vi "Serial Init.vi"(8 "error in (no error)":errorcluster, 11 "VISA Refnum in":refnum<visa-resource-name>) -> (0 "error out":errorcluster, 3 "Boolean":bool)   [LabVIEW 2017]
uses:
  <vilib>/Instr/_visa.llb/VISA Configure Serial Port (Instr).vi
  <vilib>/regexp/Match Regular Expression.xnode
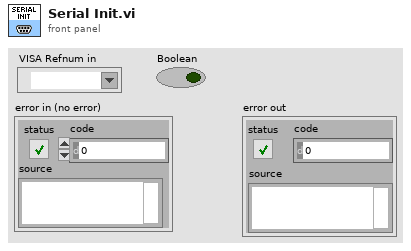
[diagram p1: front panel]
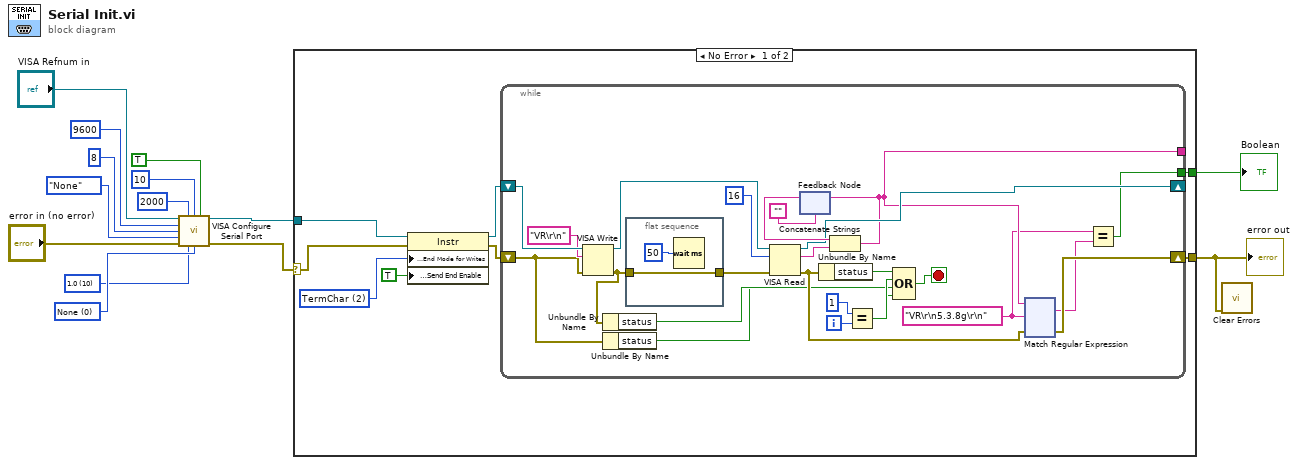
[diagram p0: block diagram]
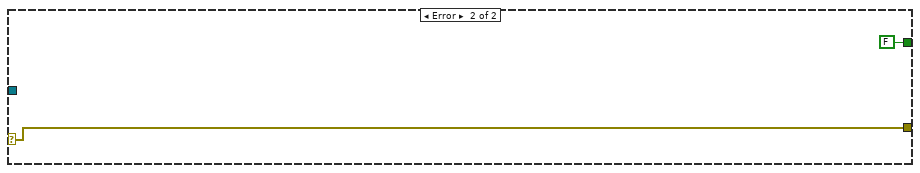
[diagram p2: hidden frame]
diagram:
  w11 = u16 0 items=["None", "XON/XOFF", "RTS/CTS", "XON/XOFF & RTS/CTS", "DTR/DSR", "XON/XOFF & DTR/DSR"] ("flow control (0:none)")
  w10 = u16 10 items=["1.0"=10, "1.5"=15, "2.0"=20] ("stop bits (10: 1 bit)")
  n1 = call-poly "VISA Configure Serial Port"("VISA resource name"="VISA Refnum in", "timeout (10sec)"=u32 2000, "termination char\n(0xA = '\\n' = LF)"=u8 10 ("termination char\n(0xA = '\\n' = LF)"), "Enable Termination\nChar (T)"=TRUE ("Enable Termination\nChar (T)"), "baud rate (9600)"=u32 9600, "data bits (8)"=u16 8, "parity (0:none)"=enum16{"None", "Odd", "Even", "Mark", "Space"}."None", "error in (no error)"="error in (no error)", "stop bits (10: 1 bit)"=w10, "flow control (0:none)"=w11) -> ("VISA resource name out"=w12:refnum<visa-resource-name>, "error out"=w1:errorcluster)  [unwired: 4 in]
  n2 = case shown="No Error" w1 {
    selector: w1 -> [w15 w163]
    tunnel: w12 -> [w22 _]
    tunnel: [w21 w163] -> w2
    tunnel: [w16 FALSE] -> w3
    frame No Error {
      w19 = u16 2 items=["None", "LastBit", "TermChar", "Break"] ("Serial Settings:Serial End Mode for Writes")
      n3 = property class="Instr"(reference=w22, error in=w15, "Serial Settings:End Mode for Writes"=w19, "Message Based Settings:Send End Enable"=TRUE) -> (reference out=w17:refnum<visa-resource-name>, error out=w18:errorcluster)
      n4 = while {
        shift-right: [w33] -> _
        shift-left: w17 -> [w46]
        shift-right: [w31] -> w21
        shift-left: w18 -> [w26]
        tunnel: [w30] -> _
        tunnel: [w28] -> w16
        i -> [w41]
        stop <- w36 stop-if-true
        w27 = "VR\r\n5.3.8g\r\n" ("x")
        n5 = VISA Write(VISA resource name=w46, write buffer="VR\r\n", error in (no error)=w26) -> (VISA resource name out=w45:refnum<visa-resource-name>, error out=w25:errorcluster)  [unwired: 1 out]
        n6 = Unbundle By Name(w25) -> ("status"=w24:bool)
        n7 = Unbundle By Name(w26) -> ("status"=w23:bool)
        n8 = flat-sequence {
          tunnel: w25 -> [w161]
          tunnel: [w161] -> w44
          frame #0 {
            n9 = Wait (ms)(milliseconds to wait=u32 50) -> ()  [unwired: 1 out]
          }
        }
        n10 = VISA Read(VISA resource name=w45, byte count=u32 16, error in (no error)=w44) -> (VISA resource name out=w33:refnum<visa-resource-name>, read buffer=w42:string, error out=w32:errorcluster)  [unwired: 1 out]
        n11 = feedback #1("") -> (w34:string)
        n12 = Unbundle By Name(w32) -> ("status"=w35:bool)
        n13 = Concatenate Strings(w34, w42) -> (w30:string)
        n14 = feedback-in #1(w30) -> ()
        n15 = Equal?(x=1, y=w41) -> (x = y?=w37:bool)
        n16 = Compound Arithmetic op=OR(w35, w37, w24, w23) -> (w36:bool)
        n17 = xnode "Match Regular Expression"("input string"=w30, "regular expression"=w27, "error in"=w32) -> ("whole match"=w29:string, "error out"=w31:errorcluster)  [unwired: 3 in, 3 out]
        n18 = Equal?(x=w27, y=w29) -> (x = y?=w28:bool)
      }
    }
    frame Error {
    }
  }
  "Boolean" <- w3
  "error out" <- w2
  n19 = call <vilib>:"Clear Errors.vi"("error in (no error)"=w2) -> ()  [unwired: 5 in, 2 out]
